vi "Perform Action.vi"(8 "error in":errorcluster, 10 "Input":variant, 11 "AI Voltage DAQmx Cont CFG in":refnum<class "AI Voltage DAQmx Cont CFG.lvclass">) -> (0 "error out":errorcluster, 2 "Output":variant, 3 "AI Voltage DAQmx Cont CFG out":refnum<class "AI Voltage DAQmx Cont CFG.lvclass">)   [LabVIEW 2023, in "AI Voltage DAQmx Cont CFG.lvclass"]
uses:
  AI Voltage DAQmx Cont CFG.lvclass
  AI Voltage DAQmx Cont CFG.lvclass/AI Voltage DAQmx Cont CFG.ctl
  DAQmx/DAQmx Base CFG/DAQmx Base CFG.lvclass
  Configuration/Configuration Semaphore/CFG Semaphore.lvclass
  b00e0f56-2a98-4529-bcc6-214aae204d95.vi
  DAQmx/DAQmx BufferLastReadsDBL/DAQmx BufferLastReadsDBL.lvclass
  DAQmx/BufferLastReadingsDBL/BufferLastReadsDBL.lvclass
  <vilib>/DAQmx/read.llb/DAQmx Read (Analog 2D DBL NChan NSamp).vi
  D:/git/HAL/HAL GOOP4/DAQmx/DAQmx BufferLastReadsDBL/DAQmx BufferLastReadsDBL.lvclass
  D:/git/HAL/HAL GOOP4/DAQmx/DAQmx Base CFG/DAQmx Base CFG.lvclass
  D:/git/HAL/HAL GOOP4/CFG Target/CFG Target.lvclass
  D:/git/HAL/HAL GOOP4/Configuration/Configuration Semaphore/CFG Semaphore.lvclass
  D:/git/HAL/HAL GOOP4/Configuration/Configuration JSON/Configuration JSON Base/CFG JSON.lvclass
  D:/git/HAL/HAL GOOP4/Interfaces/IConfigure/IConfigure.lvclass
  D:/git/HAL/HAL GOOP4/AI/AI Voltage DAQmx Cont CFG/AI Voltage DAQmx Cont CFG.lvclass
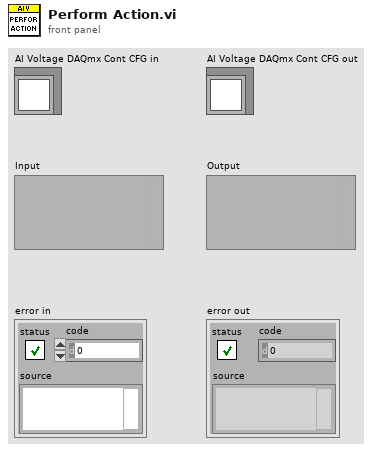
[diagram p1: front panel]
types:
  T1 = typedef "Semaphore RefNum" = refnum<k1>
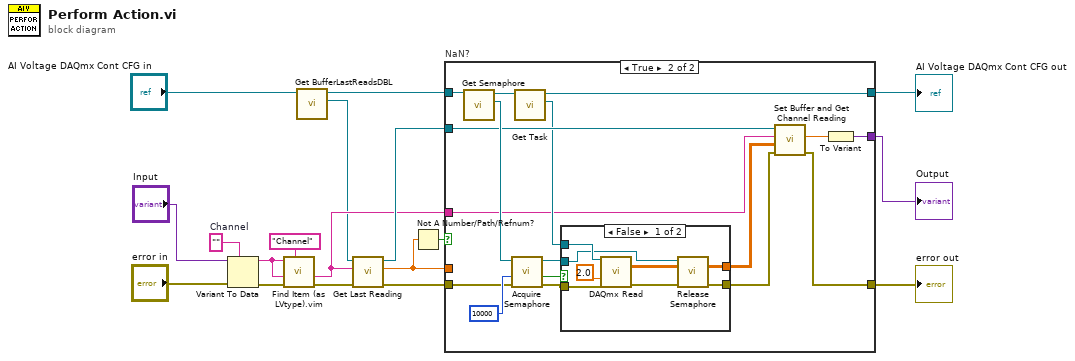
[diagram p0: block diagram]
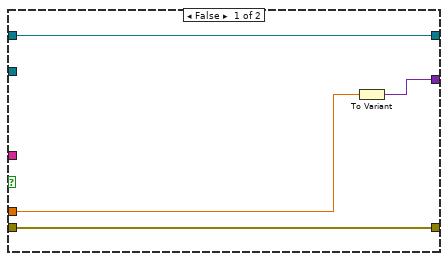
[diagram p2: hidden frame]
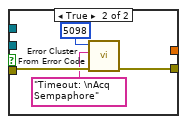
[diagram p3: hidden frame]
diagram:
  w14 = ""  # Channel
  n1 = Variant To Data(error in="error in", type=w14, Variant="Input") -> (data=w11:string, error out=w12:errorcluster)
  n2 = call "Find Item (as LVtype).vim"("$Path or Item Name"="Channel", "error in (no error)"=w12, "Data Type and Default Value"=w11, "JSON"=w11) -> ("error out"=w13:errorcluster, "Data"=w9:string)  [unwired: 4 in, 2 out]
  n3 = call "Get BufferLastReadsDBL.vi"("DAQmx BufferLastReadsDBL in"="AI Voltage DAQmx Cont CFG in") -> ("BufferLastReadsDBL.lvclass"=w7:refnum<class "BufferLastReadsDBL.lvclass">, "DAQmx BufferLastReadsDBL out"=w8:refnum<class "AI Voltage DAQmx Cont CFG.lvclass">)  [unwired: 9 in]
  n4 = call-dynamic "Get Last Reading.vi"("error in"=w13, "Channel"=w9, "BufferLastReadingsDBL in"=w7) -> ("error out"=w16:errorcluster, "Reading"=w17:dbl, "BufferLastReadingsDBL out"=w15:refnum<class "BufferLastReadsDBL.lvclass">)  [unwired: 6 in]
  n5 = Not A Number/Path/Refnum?(number/path/refnum=w17) -> (NaN/Path/Refnum?=w18:bool)
  n6 = case "NaN?" shown="True" w18 {
    tunnel: [w19 w29] -> w5
    tunnel: [w20 w23] -> w4
    tunnel: w8 -> [w20 w34]
    tunnel: w15 -> [_ w35]
    tunnel: [w21 w26] -> w1
    tunnel: w17 -> [w22 _]
    tunnel: w16 -> [w19 w28]
    tunnel: w9 -> [_ w25]
    frame False {
      n7 = To Variant(anything=w22) -> (Variant=w21:variant)
    }
    frame True {
      n8 = call "Get Semaphore.vi"("CFG Base in"=w34) -> ("Semaphore"=w39:T1, "CFG Base out"=w33:refnum<class "AI Voltage DAQmx Cont CFG.lvclass">)  [unwired: 9 in]
      n9 = call <vilib>:"Acquire Semaphore.vi"("error in (no error)"=w28, "ms timeout (-1)"=10000, "semaphore"=w39) -> ("error out"=w37:errorcluster, "timed out"=w38:bool, "semaphore out"=w27:T1)  [unwired: 2 in]
      n10 = call "Get Task.vi"("DAQmx Base CFG in"=w33) -> ("Task"=w32:refnum<k21>, "DAQmx Base CFG out"=w23:refnum<class "AI Voltage DAQmx Cont CFG.lvclass">)  [unwired: 9 in]
      n11 = case shown="False" w38 {
        tunnel: [w41 w50] -> w30
        tunnel: w37 -> [w45 w49]
        tunnel: w32 -> [w43 _]
        tunnel: [w42 _] -> w31
        tunnel: w27 -> [w40 _]
        frame False {
          n12 = call-poly <vilib>:"DAQmx Read.vi"("task/channels in"=w43, "timeout"=2.0, "error in"=w45) -> ("data"=w42:dbl[][], "error out"=w46:errorcluster)  [unwired: 10 in, 1 out]
          n13 = call <vilib>:"Release Semaphore.vi"("error in (no error)"=w46, "semaphore"=w40) -> ("error out"=w41:errorcluster)  [unwired: 4 in, 1 out]
        }
        frame True {
          n14 = call <vilib>:"Error Cluster From Error Code.vi"("error in (no error)"=w49, "error message (\"\")"="Timeout: \nAcq Sempaphore" ("error message (\"\")"), "error code (0)"=5098) -> ("error out"=w50:errorcluster)  [unwired: 6 in]
        }
      }
      n15 = call-dynamic "Set Buffer and Get Channel Reading.vi"("error in"=w30, "Readings"=w31, "Channel Ident"=w25, "BufferLastReadingsDBL in"=w35) -> ("error out"=w29:errorcluster, "Reading"=w24:dbl)  [unwired: 5 in, 1 out]
      n16 = To Variant(anything=w24) -> (Variant=w26:variant)
    }
  }
  "error out" <- w5
  "AI Voltage DAQmx Cont CFG out" <- w4
  "Output" <- w1
